vi "8-8-2 글로벌 변수.vi"() -> ()   [LabVIEW 2010]
uses:
  글로벌변수.vi
panel:
  in  "정지":bool
  out "a":dbl(graph)
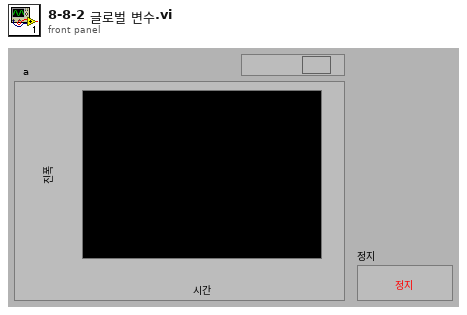
[diagram p1: front panel]
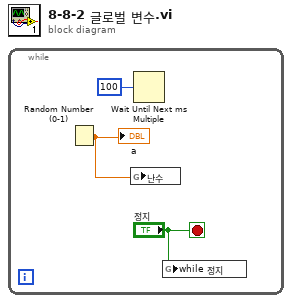
[diagram p0: block diagram]
diagram:
  n1 = while {
    stop <- "정지" stop-if-true
    n2 = Random Number (0-1)() -> (number: 0 to 1=w2:dbl)
    "a" <- w2
    n3 = global write "글로벌변수.vi" "난수"(w2) -> ()
    n4 = Wait Until Next ms Multiple(millisecond multiple=u32 100 ("ms 배수")) -> ()  [unwired: 1 out]
    n5 = global write "글로벌변수.vi" "while 정지"("정지") -> ()
  }
